vi "event_connected.vi"(11 "message":string) -> ()   [LabVIEW 2014]
uses:
  QwaveSys_ESP8266/QwaveSys_ESP8266.lvlib
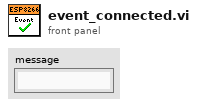
[diagram p1: front panel]
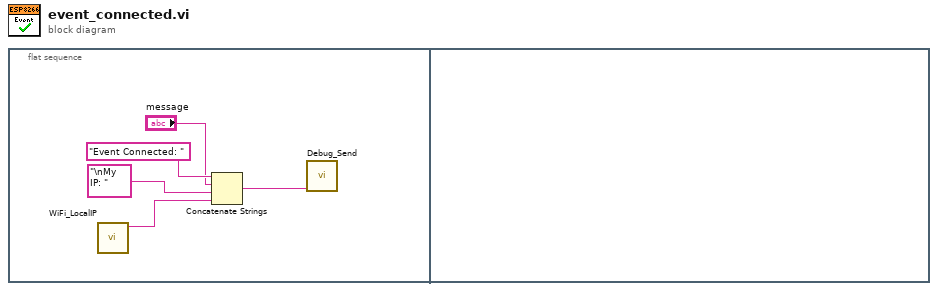
[diagram p0: block diagram]
diagram:
  n1 = flat-sequence {
    frame #0 {
      n2 = call "WiFi_LocalIP.vi"() -> ("IP"=w3:string)  [unwired: 10 in, 1 out]
      n3 = Concatenate Strings("Event Connected: " ("string"), "message", "\nMy IP: " ("string"), w3) -> (w1:string)
      n4 = call "Debug_Send.vi"("DATA"=w1) -> ()  [unwired: 11 in]
    }
    frame #1 {
    }
  }
